vi "Initialize.vi"(8 "error in (no error)":errorcluster) -> (0 "error out":errorcluster, 3 "config":T1)   [LabVIEW 2017, in "TrendAlarm.lvlib"]
uses:
  <vilib>/addons/InsightCM/Devices/Shared/Common/TrendAlarm/TrendAlarm.lvlib
  <vilib>/addons/InsightCM/Devices/Shared/Common/TrendAlarm/controls/config.ctl
  <vilib>/addons/InsightCM/Devices/Shared/Common/TrendAlarm/controls/TransitionCache.ctl
  <vilib>/addons/InsightCM/MessageBus/Base/controls/TrendAlarmTransition.ctl
  <vilib>/addons/InsightCM/Utilities/GlobalConfiguration/GlobalConfiguration.lvlib
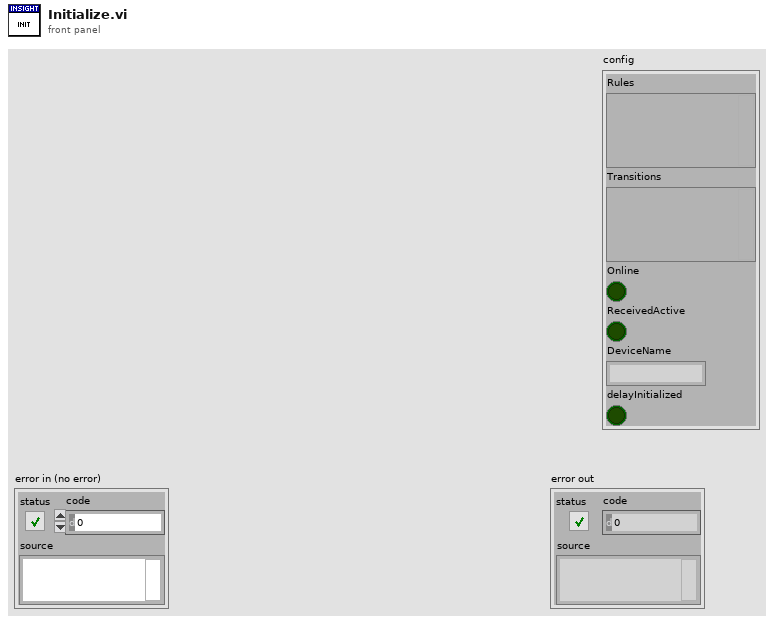
[diagram p1: front panel]
types:
  T1 = typedef "TrendAlarm.lvlib/config.ctl" = cluster{"Rules":variant, "Transitions":variant, "Online":bool, "ReceivedActive":bool, "DeviceName":string, "delayInitialized":bool}
  T2 = typedef "R2_Device.ctl" = cluster{"Id":string, "Name":string, "DeviceType":string, "HardwareName":string, "IpAddress":string, "HardwareInfo":T3[], "ApplicationType":string, "ApplicationVersion":string, "EquipmentIds":string[], "ConfigurationVersion":string, "State":T4, "Properties":T3[], "DataGroups":T5[], "BurstModeTrigger":T9}
  T3 = typedef "KeyValuePair.ctl" = cluster{"Key":string, "Value":string}
  T4 = typedef "DeviceState.ctl" = cluster{"Disabled":bool}
  T5 = typedef "R2_DataGroup.ctl" = cluster{"Name":string, "OperatingStates":T6[], "Properties":T3[], "EquipmentIds":string[], "AssetNodeId":string}
  T6 = typedef "OperatingState.ctl" = cluster{"Name":string, "Properties":T3[], "Triggers":T7[]}
  T7 = typedef "Trigger.ctl" = cluster{"Type":string, "Expression":string, "Conditions":T8[]}
  T8 = typedef "Condition.ctl" = cluster{"Source":string, "Type":string, "Operator":string, "CompareTo":string, "DwellSeconds":dbl}
  T9 = typedef "BurstModeTrigger.ctl" = cluster{"Trigger":T7, "SampleRate":string, "AcquisitionLength":string}
  T10 = typedef "AssetNode.ctl" = cluster{"Id":string, "Type":string, "Name":string, "ParentIds":string[], "State":T11, "MeasType":string, "Properties":T3[], "OperatingStates":T6[], "Metrics":T12[], "TrendAlarmRules":T13[], "References":T16[]}
  T11 = typedef "AssetState.ctl" = cluster{"Disabled":bool}
  T12 = typedef "Metric.ctl" = cluster{"Id":string, "Name":string, "Unit":string, "Properties":T3[], "MetricDefinitionInstanceId":string}
  T13 = typedef "TrendAlarmRule.ctl" = cluster{"Id":string, "AssetNodeId":string, "TrendId":string, "Disabled":bool, "OperatingState":string, "Operator":string, "Hysteresis":dbl, "OnDelaySeconds":dbl, "OffDelaySeconds":dbl, "Levels":T14[], "Properties":T3[]}
  T14 = typedef "TrendAlarmLevel.ctl" = cluster{"Severity":i32, "CompareTo":dbl, "Actions":T15[]}
  T15 = typedef "AlarmAction.ctl" = cluster{"Type":string, "Props":T3[]}
  T16 = typedef "AssetNodeReference.ctl" = cluster{"NodeId":string, "Name":string}
  T17 = typedef "TrendAlarm.lvlib/TransitionCache.ctl" = cluster{"RuleId":string, "MaxSeverity":i32, "LastTransition":T18, "OnTime":timestamp, "OffTime":timestamp}
  T18 = typedef "TrendAlarmTransition.ctl" = cluster{"At":i64, "Severity":i32, "Value":dbl}
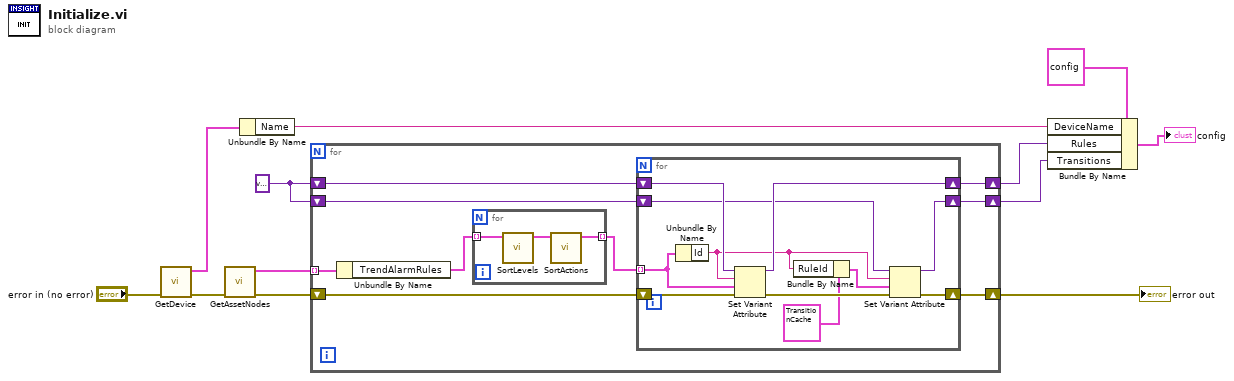
[diagram p0: block diagram]
diagram:
  w2 = variant
  n1 = call <vilib>:"GetDevice.vi"("error in (no error)"="error in (no error)") -> ("error out"=w5:errorcluster, "device configuration"=w4:T2)  [unwired: 8 in, 1 out]
  n2 = call <vilib>:"GetAssetNodes.vi"("error in (no error)"=w5) -> ("error out"=w11:errorcluster, "AssetNodes"=w12:T10[])  [unwired: 8 in, 1 out]
  n3 = Unbundle By Name(w4) -> ("Name"=w3:string)
  n4 = for {
    tunnel: w12 -> [w21] mode=indexing
    shift-right: [w18] -> w8
    shift-left: w2 -> [w17]
    shift-right: [w19] -> w10
    shift-left: w11 -> [w20]
    shift-right: [w13] -> w1
    shift-left: w2 -> [w14]
    n5 = Unbundle By Name(w21) -> ("TrendAlarmRules"=w16:T13[])
    n6 = for {
      tunnel: w16 -> [w24] mode=indexing
      tunnel: [w23] -> w15 mode=indexing
      n7 = call <vilib>:"SortLevels.vi"("rule in"=w24) -> ("rule out"=w22:T13)  [unwired: 10 in]
      n8 = call <vilib>:"SortActions.vi"("rule in"=w22) -> ("rule out"=w23:T13)  [unwired: 10 in]
    }
    n9 = for {
      tunnel: w15 -> [w32] mode=indexing
      shift-right: [w30] -> w19
      shift-left: w20 -> [w35]
      shift-right: [w34] -> w18
      shift-left: w17 -> [w33]
      shift-right: [w28] -> w13
      shift-left: w14 -> [w29]
      n10 = Unbundle By Name(w32) -> ("Id"=w25:string)
      n11 = Set Variant Attribute(Variant=w33, name=w25, value=w32, error in=w35) -> (Variant out=w34:variant, error out=w31:errorcluster)  [unwired: 1 out]
      n12 = Bundle By Name(cluster=T17 {"RuleId"="", "MaxSeverity"=0, "LastTransition"={"At"=0, "Severity"=0, "Value"=0.0}, "OnTime"=timestamp(0 s since 1904-01-01), "OffTime"=timestamp(0 s since 1904-01-01)} ("cache out"), "RuleId"=w25) -> (w26:T17)
      n13 = Set Variant Attribute(Variant=w29, name=w25, value=w26, error in=w31) -> (Variant out=w28:variant, error out=w30:errorcluster)  [unwired: 1 out]
    }
  }
  "error out" <- w10
  n14 = Bundle By Name(cluster=T1 {"Rules"=variant, "Transitions"=variant, "Online"=FALSE, "ReceivedActive"=FALSE, "DeviceName"="", "delayInitialized"=FALSE} ("config"), "DeviceName"=w3, "Rules"=w8, "Transitions"=w1) -> (→"config":T1)
